vi "Save Plot Data.vi"(8 "error in":errorcluster, 10 "XY Graph":cluster{i32[], i32[]}[](array[cluster]), 11 "XYGraph in":refnum<vi>) -> (0 "error out":errorcluster)   [LabVIEW 2017, in "DTacq Plot Display Library.lvlib"]
uses:
  DTacq Plot Display Library.lvlib
  <vilib>/Utility/file.llb/Write Delimited Spreadsheet (string).vi
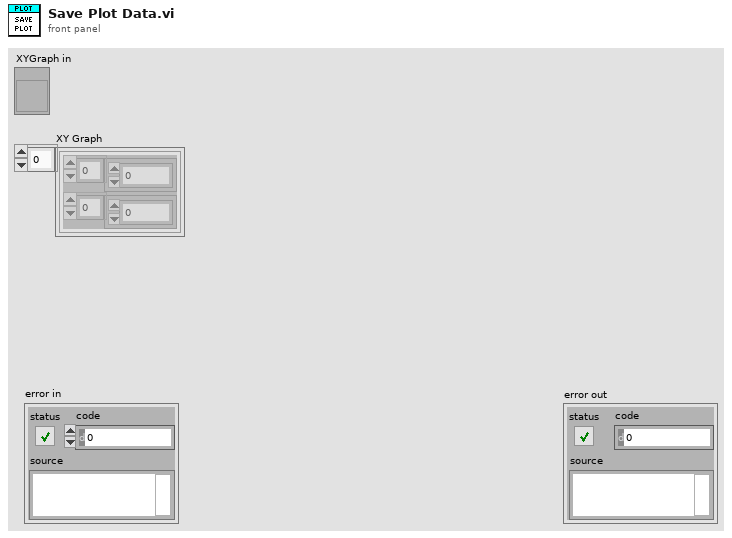
[diagram p1: front panel]
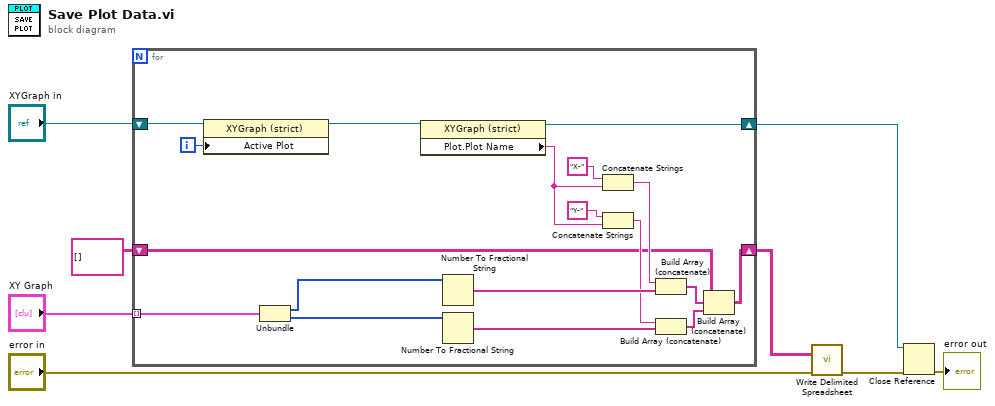
[diagram p0: block diagram]
diagram:
  n1 = for {
    tunnel: "XY Graph" -> [w23] mode=indexing
    shift-right: [w11] -> w6
    shift-left: string[][] [] -> [w10]
    shift-right: [w9] -> w2
    shift-left: "XYGraph in" -> [w26]
    i -> [w25]
    n2 = property class="XYGraph (strict)"(reference=w26, "Active Plot"=w25) -> (reference out=w24:refnum<vi>)  [unwired: 1 in, 1 out]
    n3 = Unbundle(w23) -> (w22:i32[], w21:i32[])
    n4 = property class="XYGraph (strict)"(reference=w24) -> (reference out=w9:refnum<vi>, "Plot.Plot Name"=w18:string)  [unwired: 1 in, 1 out]
    n5 = Number To Fractional String(number=w22) -> (F-format string=w17:string[])  [unwired: 3 in]
    n6 = Number To Fractional String(number=w21) -> (F-format string=w15:string[])  [unwired: 3 in]
    n7 = Concatenate Strings("X-" ("string"), w18) -> (w16:string)
    n8 = Concatenate Strings("Y-" ("string"), w18) -> (w14:string)
    n9 = Build Array (concatenate)(w16, w17) -> (w12:string[])
    n10 = Build Array (concatenate)(w14, w15) -> (w13:string[])
    n11 = Build Array (concatenate)(w10, w12, w13) -> (w11:string[][])
  }
  n12 = call-poly <vilib>:"Write Delimited Spreadsheet.vi"("2D data"=w6, "error in (no error)"="error in") -> ("error out"=w3:errorcluster)  [unwired: 12 in, 1 out]
  n13 = Close Reference(reference=w2, error in (no error)=w3) -> (error out=→"error out":errorcluster)
